vi "Get USB Strings.vi"(6 "error in (no error)":errorcluster, 9 "DeviceRefnum":u64) -> (0 "error out":errorcluster, 2 "Device USB Strings":T1, 3 "DeviceRefnum Out":u64)   [LabVIEW 2016]
doc: "Get USB device strings."
panel:
  in  "serial":string
  in  "product":string
  in  "manufact":string
  out "function return":i32
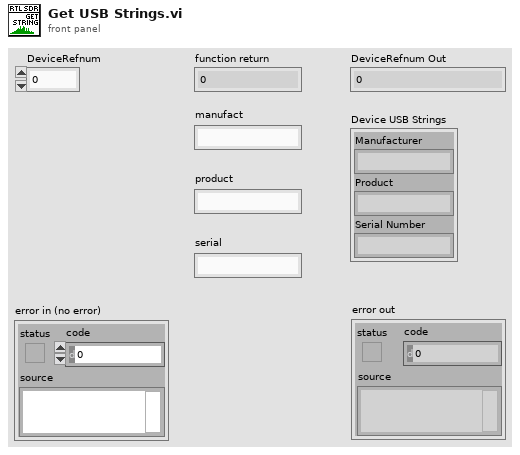
[diagram p1: front panel]
types:
  T1 = cluster{"Manufacturer":string, "Product":string, "Serial Number":string}
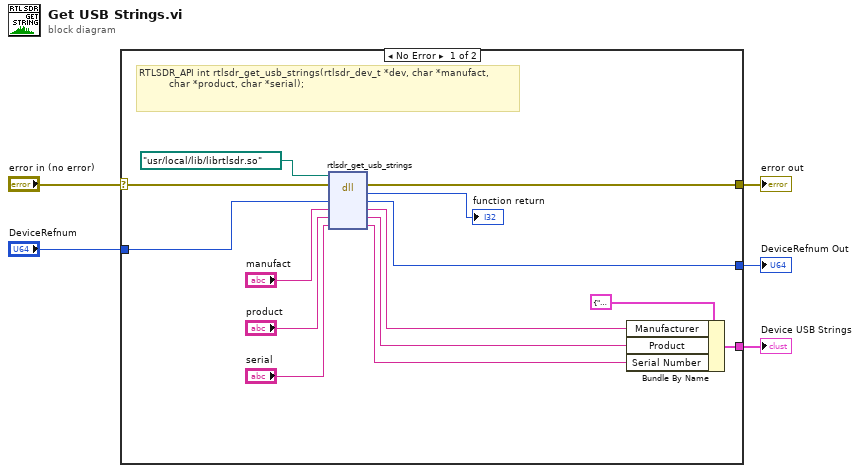
[diagram p0: block diagram]
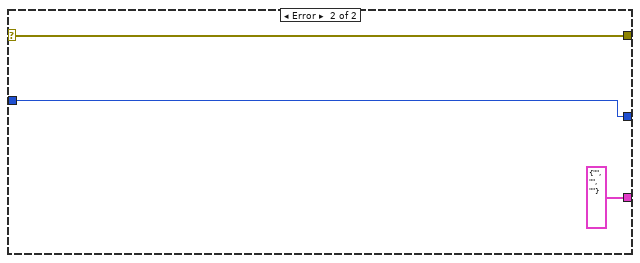
[diagram p2: hidden frame]
diagram:
  n1 = case shown="No Error" "error in (no error)" {
    selector: "error in (no error)" -> [w7 w22]
    tunnel: [w15 w22] -> w5
    tunnel: [w13 T1 {"Manufacturer"="", "Product"="", "Serial Number"=""}] -> w4
    tunnel: "DeviceRefnum" -> [w8 w21]
    tunnel: [w6 w21] -> w1
    frame No Error {
      # "RTLSDR_API int rtlsdr_get_usb_strings(rtlsdr_dev_t *dev, char *manufact,\n\t\t\t\t      char *product, char *serial);"
      n2 = dll-call lib="C:/Program Files (x86)/National Instruments/LabVIEW 2016/user.lib/rtlsdr/rtlsdr.*" fn="rtlsdr_get_usb_strings"(path in=path "/usr/local/lib/librtlsdr.so", error in=w7, "DeviceRefnum"=w8, "manufact"="manufact", "product"="product", "serial"="serial") -> (error out=w15:errorcluster, "return type"=→"function return":i32, "DeviceRefnum"=w6:u64, "manufact"=w12:string, "product"=w11:string, "serial"=w10:string)  [unwired: 1 in, 1 out]
      n3 = Bundle By Name(cluster=T1 {"Manufacturer"="", "Product"="", "Serial Number"=""}, "Manufacturer"=w12, "Product"=w11, "Serial Number"=w10) -> (w13:T1)
    }
    frame Error {
    }
  }
  "error out" <- w5
  "Device USB Strings" <- w4
  "DeviceRefnum Out" <- w1
